vi "Post-Init.vi"(8 "error in (no error)":errorcluster, 11 "Instrument Driver in":refnum<class "Instrument Driver.lvclass">) -> (0 "error out":errorcluster, 2 "Init Result":refnum<class "Acquired Result.lvclass">, 3 "Instrument Driver out":refnum<class "Instrument Driver.lvclass">)   [LabVIEW 2019, in "Instrument Driver.lvclass"]
uses:
  Instrument Driver.lvclass
  Results/Start Stream Result/Start Stream Result.lvclass
  Results/Acquired Result/Acquired Result.lvclass
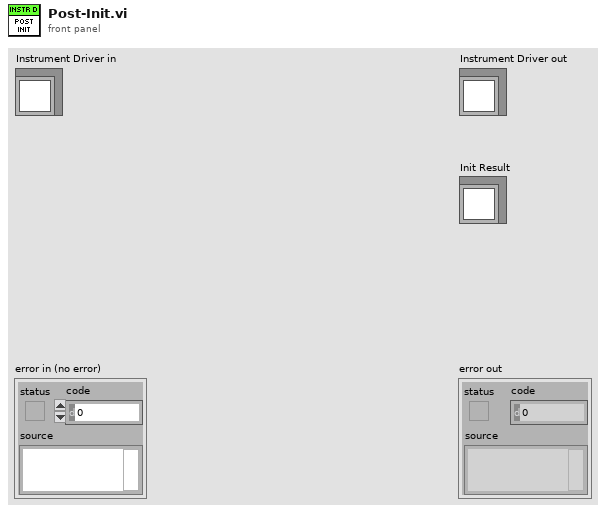
[diagram p1: front panel]
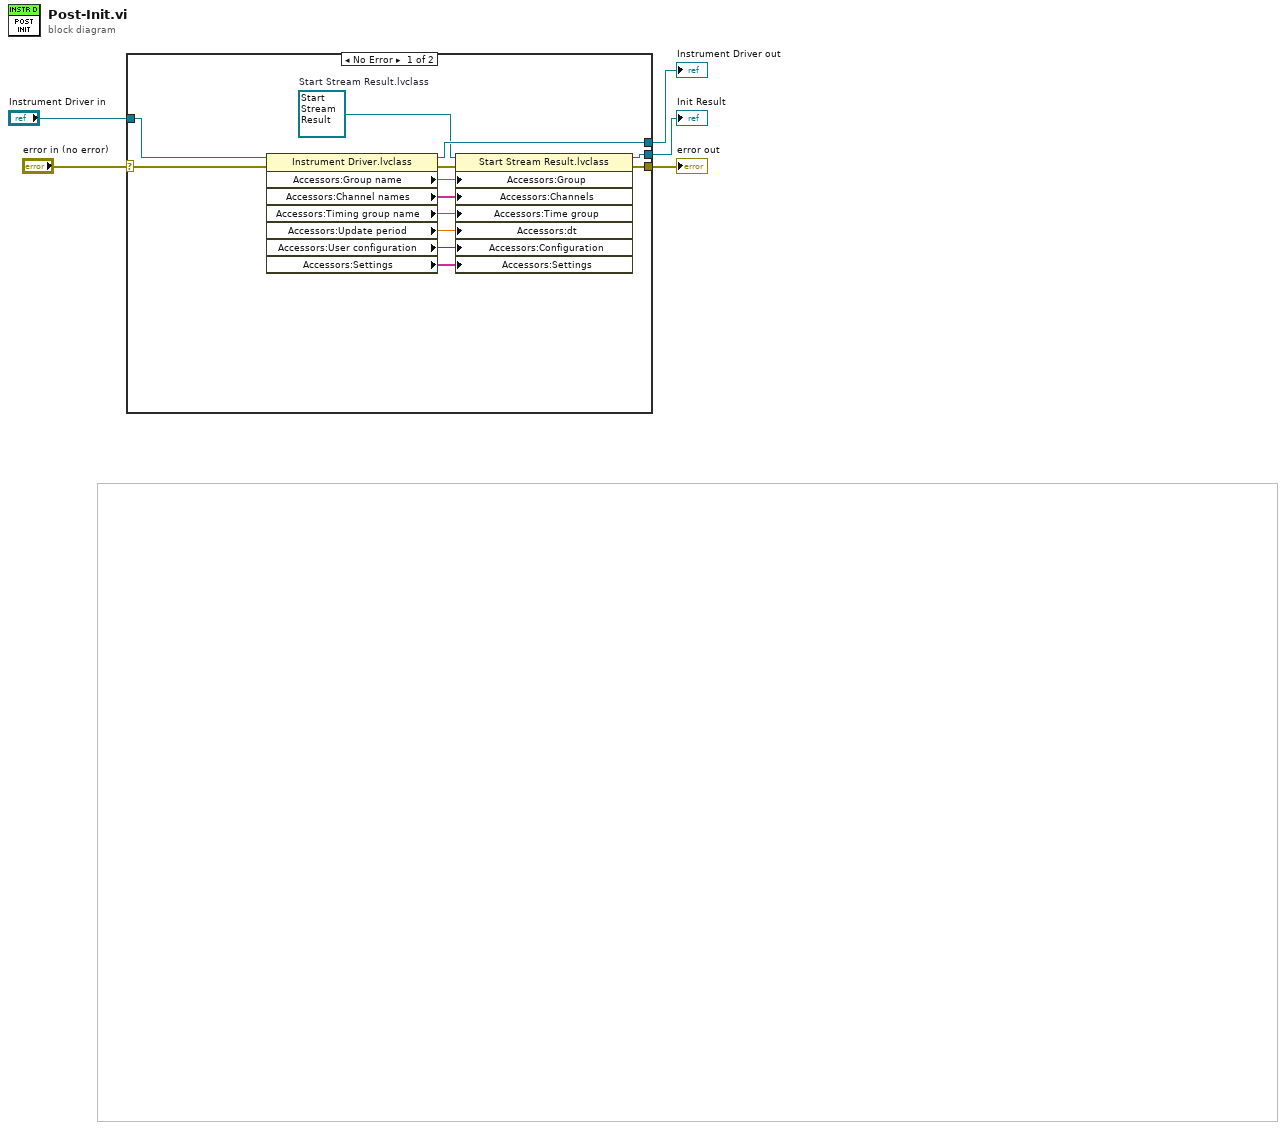
[diagram p0: block diagram]
diagram:
  n1 = case shown="No Error" "error in (no error)" {
    selector: "error in (no error)" -> [w18 w20]
    tunnel: [w12 w20] -> w4
    tunnel: [w16 w19] -> w2
    tunnel: "Instrument Driver in" -> [w17 w19]
    tunnel: [w11 _] -> w1
    frame No Error {
      w15 = refnum<class "Start Stream Result.lvclass"> refnum  # Start Stream Result.lvclass
      n2 = property class="Instrument Driver.lvclass"(reference=w17, error in=w18) -> (reference out=w16:refnum<class "Instrument Driver.lvclass">, error out=w13:errorcluster, "Accessors:Group name"=w14:string, "Accessors:Channel names"=w7:string[], "Accessors:Timing group name"=w8:string, "Accessors:Update period"=w9:dbl, "Accessors:User configuration"=w10:variant, "Accessors:Settings"=w6:string[])
      n3 = property class="Start Stream Result.lvclass"(reference=w15, error in=w13, "Accessors:Group"=w14, "Accessors:Channels"=w7, "Accessors:Time group"=w8, "Accessors:dt"=w9, "Accessors:Configuration"=w10, "Accessors:Settings"=w6) -> (reference out=w11:refnum<class "Start Stream Result.lvclass">, error out=w12:errorcluster)
    }
    frame Error {
    }
  }
  "error out" <- w4
  "Instrument Driver out" <- w2
  "Init Result" <- w1
